vi "Save QD suggestions.vi"(8 "error in":errorcluster, 10 "Position":T1, 11 "Suggestions":cluster{"Class Name":string, "Count":i32}[](array[cluster])) -> (0 "error out":errorcluster)   [LabVIEW 2024]
uses:
  <vilib>/Utility/miscctls.llb/LVPositionTypeDef.ctl
  QD Data.ctl
  QD Suggestion.ctl
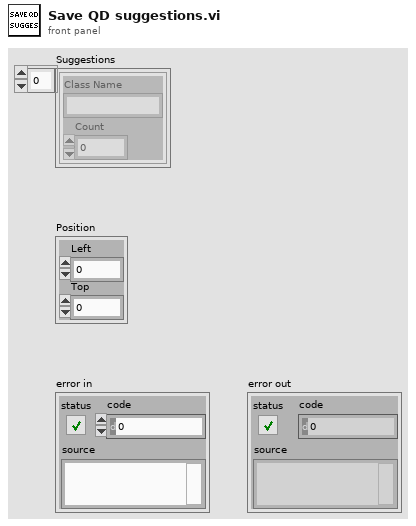
[diagram p1: front panel]
types:
  T1 = typedef "LVPositionTypeDef.ctl" = cluster{"Left":i32, "Top":i32}
  T2 = typedef "QD Data.ctl" = cluster{T3[], cluster{"Left":i32, "Top":i32}}
  T3 = typedef "QD Suggestion.ctl" = cluster{"Data":string, "qd":string[], "Type":string}
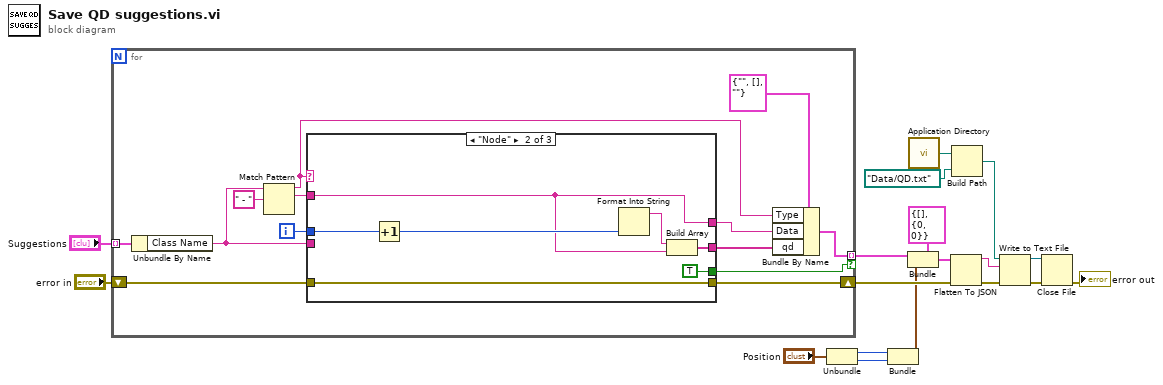
[diagram p0: block diagram]
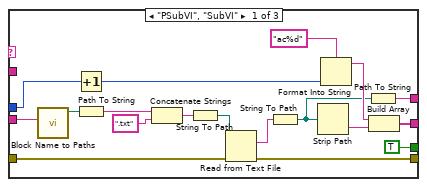
[diagram p2: hidden frame]
diagram:
  n1 = for {
    tunnel: "Suggestions" -> [w31] mode=indexing
    tunnel: [w28] -> w10 mode=indexing if=w25
    shift-right: [w21] -> w12
    shift-left: "error in" -> [w22]
    i -> [w26]
    n2 = Unbundle By Name(w31) -> ("Class Name"=w20:string)
    n3 = Match Pattern(string=w20, regular expression=" - " ("search string/char (-)")) -> (before substring=w19:string, match substring=w29:string)  [unwired: 1 in, 2 out]
    n4 = case shown="\"Node\"" w19 {
      tunnel: [TRUE ("Boolean") TRUE ("Boolean") _] -> w25
      tunnel: w29 -> [_ w50 _]
      tunnel: w20 -> [w44 _ _]
      tunnel: [w37 w53 _] -> w27
      tunnel: w26 -> [w36 w52 _]
      tunnel: [w35 w50 _] -> w24
      tunnel: w22 -> [w34 w51 w57]
      tunnel: [w33 w51 w57] -> w21
      frame "PSubVI", "SubVI" {
        n5 = call "Block Name to Paths.vi"("Block Name"=w44) -> ("Block Path"=w45:path)  [unwired: 9 in, 1 out]
        n6 = Increment(x=w36) -> (x+1=w41:i32)
        n7 = Path To String(path=w45) -> (string=w49:string)
        n8 = Concatenate Strings(w49, ".txt" ("string")) -> (w47:string)
        n9 = String To Path(string=w47) -> (path=w43:path)
        n10 = Read from Text File(file (use dialog)=w43, error in=w34) -> (text=w46:string, error out=w33:errorcluster)  [unwired: 2 in, 2 out]
        n11 = String To Path(string=w46) -> (path=w32:path)
        n12 = Strip Path(path=w32) -> (name=w38:string)  [unwired: 1 out]
        n13 = Format Into String(format string="ac%d", w41) -> (resulting string=w39:string)  [unwired: 2 in, 1 out]
        n14 = Path To String(path=w32) -> (string=w35:string)
        n15 = Build Array(w39, w38) -> (w37:string[])
      }
      frame "Node" {
        n16 = Increment(x=w52) -> (x+1=w55:i32)
        n17 = Format Into String(w55) -> (resulting string=w54:string)  [unwired: 3 in, 1 out]
        n18 = Build Array(w54, w50) -> (w53:string[])
      }
      frame Default {
      }
    }
    n19 = Bundle By Name(cluster=T3 {"Data"="", "qd"=[], "Type"=""}, "Type"=w19, "Data"=w24, "qd"=w27) -> (w28:T3)
  }
  n20 = Unbundle("Position") -> ("Left"=w8:i32, "Top"=w7:i32)
  n21 = Bundle("Left"=w8, "Top"=w7) -> (w6:cluster{"Left":i32, "Top":i32})  [unwired: 1 in]
  n22 = Bundle(cluster=T2 {[], {"Left"=0, "Top"=0}}, w10, w6) -> (w5:T2)
  n23 = call <vilib>:"Application Directory.vi"() -> ("Application Directory"=w3:path)
  n24 = Flatten To JSON(anything=w5, error in (no error)=w12) -> (JSON string=w16:string, 11:w17:errorcluster)  [unwired: 1 in]
  n25 = Build Path(base path=w3, name or relative path=path "Data/QD.txt" ("file (use dialog)")) -> (appended path=w1:path)
  n26 = Write to Text File(file (use dialog)=w1, text=w16, error in=w17) -> (refnum out=w15:refnum<file>, error out=w14:errorcluster)  [unwired: 1 in, 1 out]
  n27 = Close File(refnum=w15, error in=w14) -> (error out=→"error out":errorcluster)  [unwired: 1 out]
